vi "Save_QPT_Data_Main_v2.vi"(7 "Numeric":u32, 8 "error in":errorcluster, 9 "Save CYCLOPS data (?)":bool, 10 "Save raw data (?)":bool, 11 "Data Raw":dbl[][](array[numeric])) -> (0 "error out":errorcluster, 3 "Data CYCLOPS":dbl[][](array[numeric]))   [LabVIEW 2021]
uses:
  <vilib>/Utility/file.llb/Write Delimited Spreadsheet (DBL).vi
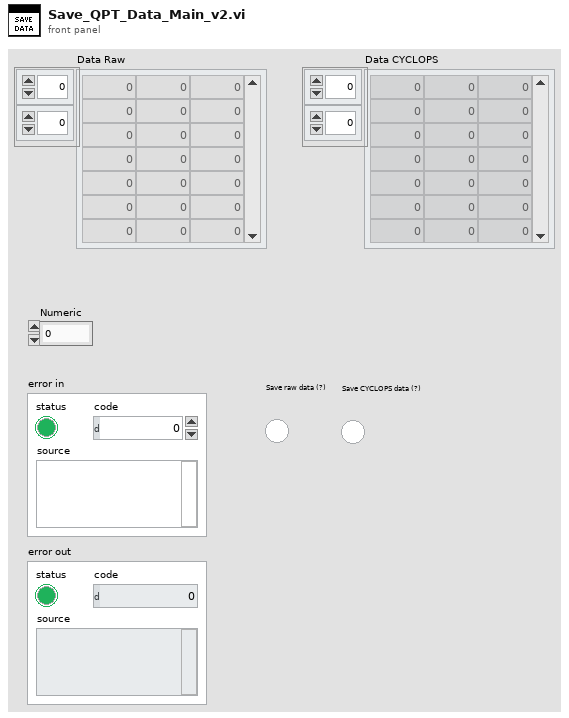
[diagram p1: front panel]
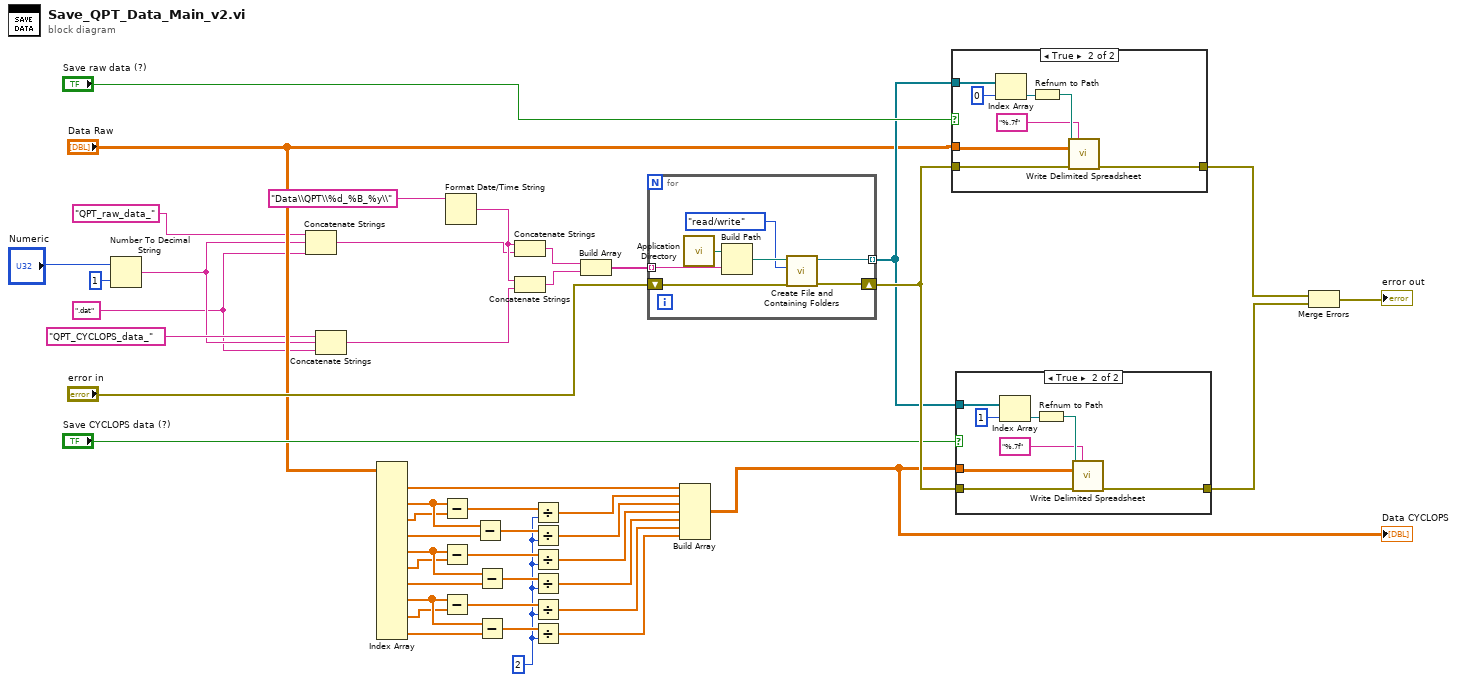
[diagram p0: block diagram]
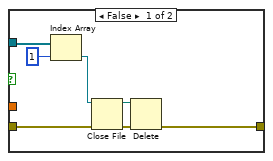
[diagram p2: hidden frame]
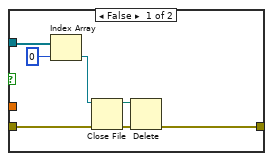
[diagram p3: hidden frame]
diagram:
  w2 = ".dat"
  w17 = 2
  n1 = Number To Decimal String(number="Numeric", width (-)=i16 1) -> (decimal integer string=w3:string)
  n2 = Concatenate Strings("QPT_raw_data_", w3, w2) -> (w5:string)
  n3 = Concatenate Strings("QPT_CYCLOPS_data_", w3, w2) -> (w1:string)
  n4 = Index Array(array="Data Raw") -> (element #1=w32:dbl[], element #2=w31:dbl[], element #3=w30:dbl[], element #4=w33:dbl[], element #5=w29:dbl[], element #6=w28:dbl[], element #7=w27:dbl[], element #8=w26:dbl[], element #9=w24:dbl[], element #10=w25:dbl[])  [unwired: 20 in]
  n5 = Subtract(x=w31, y=w30) -> (x-y=w23:dbl[])
  n6 = Subtract(x=w29, y=w28) -> (x-y=w19:dbl[])
  n7 = Subtract(x=w26, y=w24) -> (x-y=w21:dbl[])
  n8 = Format Date/Time String(time format string (%c)="Data\\QPT\\%d_%B_%y\\") -> (date/time string=w9:string)  [unwired: 2 in]
  n9 = Subtract(x=w31, y=w33) -> (x-y=w22:dbl[])
  n10 = Subtract(x=w29, y=w27) -> (x-y=w18:dbl[])
  n11 = Subtract(x=w26, y=w25) -> (x-y=w20:dbl[])
  n12 = Concatenate Strings(w9, w5) -> (w46:string)
  n13 = Concatenate Strings(w9, w1) -> (w45:string)
  n14 = Divide(x=w23, y=w17) -> (x/y=w11:dbl[])
  n15 = Divide(x=w22, y=w17) -> (x/y=w12:dbl[])
  n16 = Divide(x=w19, y=w17) -> (x/y=w13:dbl[])
  n17 = Divide(x=w18, y=w17) -> (x/y=w14:dbl[])
  n18 = Divide(x=w21, y=w17) -> (x/y=w15:dbl[])
  n19 = Divide(x=w20, y=w17) -> (x/y=w16:dbl[])
  n20 = Build Array(w46, w45) -> (w44:string[])
  n21 = for {
    tunnel: [w47] -> w40 mode=indexing
    tunnel: w44 -> [w50] mode=indexing
    shift-right: [w48] -> w41
    shift-left: "error in" -> [w49]
    n22 = call <vilib>:"Application Directory.vi"() -> ("Application Directory"=w52:path)
    n23 = Build Path(base path=w52, name or relative path=w50) -> (appended path=w53:path)
    n24 = call <vilib>:"Create File and Containing Folders.vi"("error in (no error)"=w49, "access"=enum16{"read/write", "read-only", "write-only"}."read/write", "file path"=w53) -> ("error out"=w48:errorcluster, "refnum out"=w47:refnum<file>)  [unwired: 7 in]
  }
  n25 = Build Array(w32, w11, w12, w13, w14, w15, w16) -> (w34:dbl[][])
  "Data CYCLOPS" <- w34
  n26 = case shown="True" "Save raw data (?)" {
    tunnel: w40 -> [w59 w67]
    tunnel: "Data Raw" -> [_ w66]
    tunnel: w41 -> [w55 w65]
    tunnel: [w58 w64] -> w39
    frame False {
      n27 = Index Array(array=w59, index=0) -> (element=w56:refnum<file>)
      n28 = Close File(refnum=w56, error in=w55) -> (path=w57:path, error out=w54:errorcluster)
      n29 = Delete(path (use dialog)=w57, error in=w54) -> (error out=w58:errorcluster)  [unwired: 3 in, 2 out]
    }
    frame True {
      n30 = Index Array(array=w67, index=0) -> (element=w63:refnum<file>)
      n31 = Refnum to Path(1:w63) -> (0:w62:path)
      n32 = call-poly <vilib>:"Write Delimited Spreadsheet.vi"("file path (dialog if empty)"=w62, "format (%.3f)"="%.7f", "2D data"=w66, "error in (no error)"=w65) -> ("error out"=w64:errorcluster)  [unwired: 10 in, 1 out]
    }
  }
  n33 = case shown="True" "Save CYCLOPS data (?)" {
    tunnel: w40 -> [w74 w82]
    tunnel: w34 -> [_ w81]
    tunnel: w41 -> [w70 w80]
    tunnel: [w73 w79] -> w38
    frame False {
      n34 = Index Array(array=w74, index=1) -> (element=w71:refnum<file>)
      n35 = Close File(refnum=w71, error in=w70) -> (path=w72:path, error out=w69:errorcluster)
      n36 = Delete(path (use dialog)=w72, error in=w69) -> (error out=w73:errorcluster)  [unwired: 3 in, 2 out]
    }
    frame True {
      n37 = Index Array(array=w82, index=1) -> (element=w78:refnum<file>)
      n38 = Refnum to Path(1:w78) -> (0:w77:path)
      n39 = call-poly <vilib>:"Write Delimited Spreadsheet.vi"("file path (dialog if empty)"=w77, "format (%.3f)"="%.7f", "2D data"=w81, "error in (no error)"=w80) -> ("error out"=w79:errorcluster)  [unwired: 10 in, 1 out]
    }
  }
  n40 = Merge Errors(w39, w38) -> (→"error out":errorcluster)
